vi "LoggingLoop.vi"(8 "Error In":errorcluster, 11 "Communication References":T1) -> (0 "Error Out":errorcluster)   [LabVIEW 2017, in "Client.lvlib" / "ClientLogger.lvlib"]
doc: "This Loop accepts \"Log\"-Messages with LogData.ctl as Datatype. It then logs the Type of Message, the Message Data and the Timestamp of the message to a tdms-file."
uses:
  ClientLogger.lvlib
  CommunicationsFrameWork/TypeDefs/CommReferences.ctl
  CommunicationsFrameWork/TypeDefs/MessageCluster.ctl
  TypeDefs/LoggingLoopData.ctl
  TypeDefs/LogData.ctl
  <vilib>/Utility/error.llb/Error Cluster From Error Code.vi
  <vilib>/ErrorRing/Error Ring.xnode
  ClientErrorHandler/ClientErrorHandler.lvlib
  CommunicationsFrameWork/CommsFrameWork.lvlib
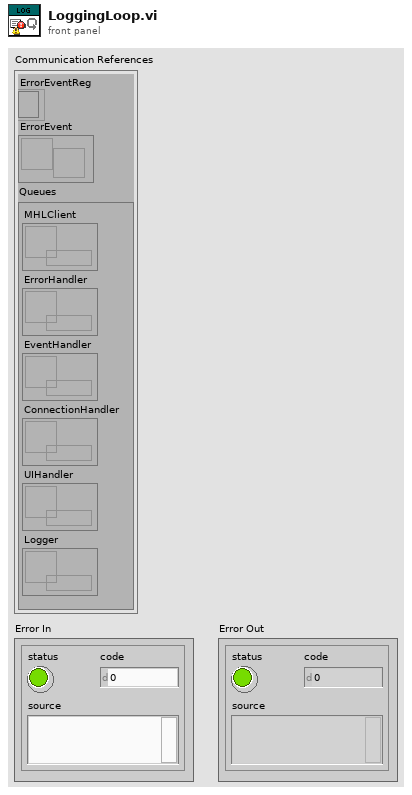
[diagram p1: front panel]
types:
  T1 = typedef "Client.lvlib/CommsFrameWork.lvlib/CommReferences.ctl" = cluster{"ErrorEventReg":refnum<event-registration>, "ErrorEvent":refnum<user-event>, "Queues":cluster{"MHLClient":refnum<queue>, "ErrorHandler":refnum<queue>, "EventHandler":refnum<queue>, "ConnectionHandler":refnum<queue>, "UIHandler":refnum<queue>, "Logger":refnum<queue>}}
  T2 = typedef "Client.lvlib/ClientLogger.lvlib/LoggingLoopData.ctl" = cluster{"TDMS Ref":refnum<k34>, "LogPath":path}
  T3 = enum16{"open", "open or create", "create or replace", "create", "open (read-only)"}
  T4 = typedef "Client.lvlib/ClientLogger.lvlib/LogData.ctl" = cluster{"Time":timestamp, "Type":string, "LogText":string}
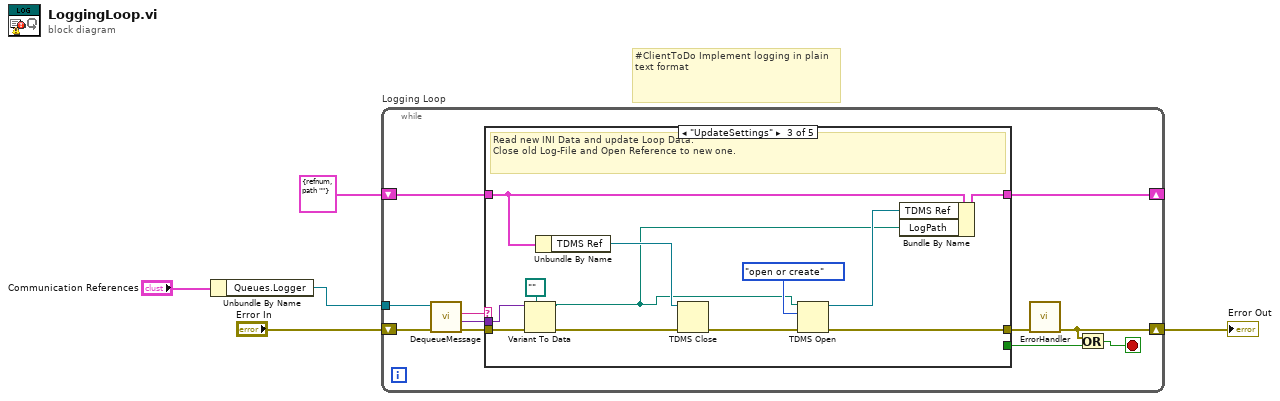
[diagram p0: block diagram]
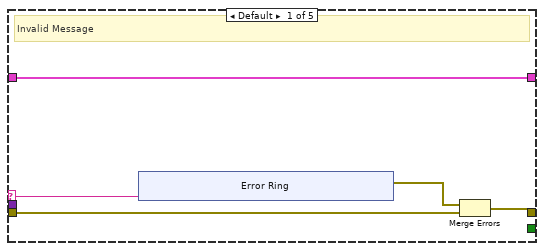
[diagram p2: hidden frame]
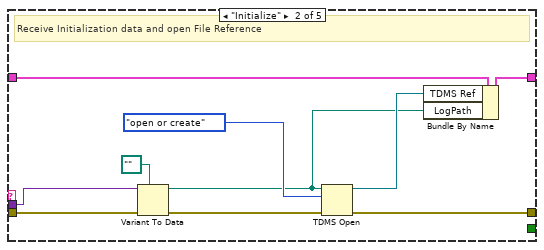
[diagram p3: hidden frame]
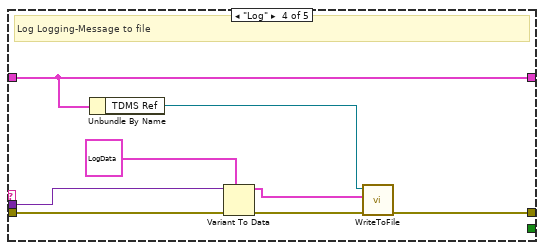
[diagram p4: hidden frame]
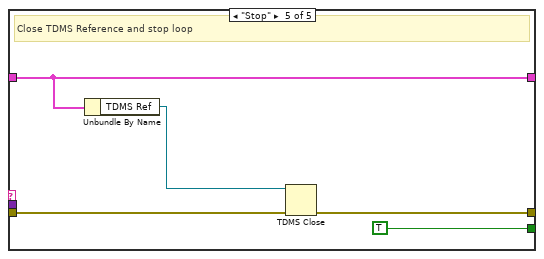
[diagram p5: hidden frame]
diagram:
  # "#ClientToDo Implement logging in plain text format"
  n1 = Unbundle By Name("Communication References") -> ("Queues.Logger"=w3:refnum<queue>)
  n2 = while "Logging Loop" {
    shift-right: [w11] -> w4
    shift-left: "Error In" -> [w9]
    tunnel: w3 -> [w10]
    shift-right: [w14] -> _
    shift-left: T2 {"TDMS Ref"=refnum, "LogPath"=path ""} ("LoggingLoopData") -> [w15]
    stop <- w13 stop-if-true
    n3 = call "DequeueMessage.vi"("error in (no error)"=w9, "Message Queue"=w10) -> ("error out"=w8:errorcluster, "Message Data"=w6:variant, "Message"=w7:string)  [unwired: 5 in, 2 out]
    n4 = case shown="\"UpdateSettings\"" w7 {
      selector: w7 -> [w20 _ _ _ _]
      tunnel: [w19 w37 w49 w54 w61] -> w12
      tunnel: w8 -> [w21 w38 w50 w58 w63]
      tunnel: w6 -> [_ w33 w46 w56 _]
      tunnel: [_ _ _ _ TRUE] -> w16
      tunnel: [w17 w32 w45 w52 w60] -> w14
      tunnel: w15 -> [w17 w35 w43 w52 w60]
      frame Default {
        # "Invalid Message"
        n5 = xnode "Error Ring"("parameter 0"=w20) -> ("error out"=w18:errorcluster)
        n6 = Merge Errors(w18, w21) -> (w19:errorcluster)
      }
      frame "Initialize" {
        # "Receive Initialization data and open File Reference"
        n7 = Variant To Data(error in=w38, type=path "", Variant=w33) -> (data=w29:path, error out=w34:errorcluster)
        n8 = TDMS Open(8:w34, 10:T3."open or create" ("operation (0:open)"), 11:w29) -> (0:w37:errorcluster, 3:w31:refnum<k34>)  [unwired: 4 in]
        n9 = Bundle By Name(cluster=w35, "TDMS Ref"=w31, "LogPath"=w29) -> (w32:T2)
      }
      frame "UpdateSettings" {
        # "Read new INI Data and update Loop Data.\nClose old Log-File and Open Reference to new one."
        n10 = Variant To Data(error in=w50, type=path "", Variant=w46) -> (data=w39:path, error out=w47:errorcluster)
        n11 = Unbundle By Name(w43) -> ("TDMS Ref"=w41:refnum<k34>)
        n12 = TDMS Close(8:w47, 11:w41) -> (0:w42:errorcluster)  [unwired: 1 out]
        n13 = TDMS Open(8:w42, 10:T3."open or create" ("operation (0:open)"), 11:w39) -> (0:w49:errorcluster, 3:w44:refnum<k34>)  [unwired: 4 in]
        n14 = Bundle By Name(cluster=w43, "TDMS Ref"=w44, "LogPath"=w39) -> (w45:T2)
      }
      frame "Log" {
        # "Log Logging-Message to file"
        n15 = Unbundle By Name(w52) -> ("TDMS Ref"=w51:refnum<k34>)
        n16 = Variant To Data(error in=w58, type=T4 {"Time"=timestamp(0 s since 1904-01-01), "Type"="", "LogText"=""} ("LogData"), Variant=w56) -> (data=w53:T4, error out=w57:errorcluster)
        n17 = call "WriteToFile.vi"("error in (no error)"=w57, "LogData"=w53, "Refnum in"=w51) -> ("error out"=w54:errorcluster)  [unwired: 7 in, 1 out]
      }
      frame "Stop" {
        # "Close TDMS Reference and stop loop"
        n18 = Unbundle By Name(w60) -> ("TDMS Ref"=w59:refnum<k34>)
        n19 = TDMS Close(8:w63, 11:w59) -> (0:w61:errorcluster)  [unwired: 1 out]
      }
    }
    n20 = call "ErrorHandler.vi"("error in (no error)"=w12) -> ("error out"=w11:errorcluster)  [unwired: 10 in]
    n21 = Or(x=w11, y=w16) -> (x .or. y?=w13:bool)
  }
  "Error Out" <- w4
